vi "模字量AD输入统计结果.vi"   [LabVIEW 2010]
uses:
  全局量/自动测试结果.vi
  全局量/全局_配置.vi
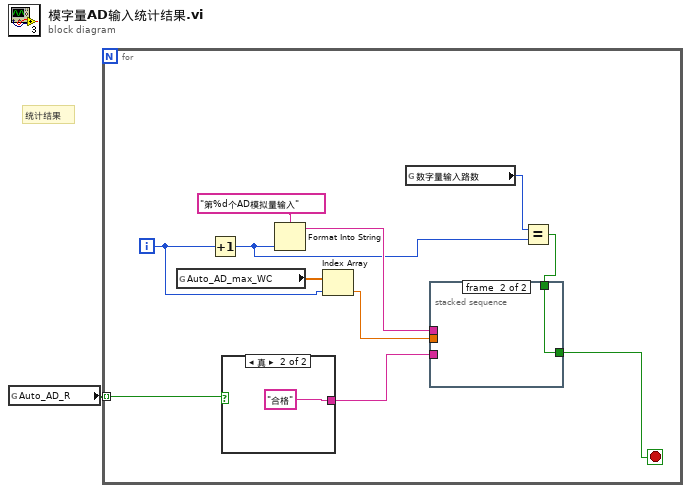
[diagram p0: block diagram]
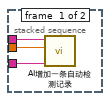
[diagram p2: hidden frame]
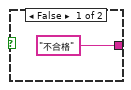
[diagram p3: hidden frame]
diagram:
  # "统计结果"
  n1 = global read "自动测试结果.vi" "Auto_AD_R"() -> (w1:bool[])
  n2 = for {
    tunnel: w1 -> [w12] mode=indexing
    i -> [w7]
    stop <- w3 stop-if-true
    n3 = global read "自动测试结果.vi" "Auto_AD_max_WC"() -> (w8:dbl[])
    n4 = Increment(x=w7) -> (x+1=w4:i32)
    n5 = case shown="真" w12 {
      tunnel: ["不合格" "合格"] -> w9
      frame False {
      }
      frame True {
      }
    }
    n6 = Format Into String(format string="第%d个AD模拟量输入", w4) -> (resulting string=w10:string)  [unwired: 2 in, 1 out]
    n7 = Index Array(array=w8, index=w7) -> (element=w6:dbl)
    n8 = global read "全局_配置.vi" "数字量输入路数"() -> (w5:i32)
    n9 = Equal?(x=w5, y=w4) -> (x = y?=w2:bool)
    n10 = stacked-sequence {
      tunnel: w10 -> [w15 _]
      tunnel: w9 -> [w14 _]
      tunnel: w6 -> [w13 _]
      tunnel: [_ w16] -> w3
      tunnel: w2 -> [_ w16]
      frame #0 {
        n11 = call "AI增加一条自动检测记录.vi"("测试结果"=w14, "最大误差"=w13, "测试内容"=w15) -> ()  [unwired: 9 in]
      }
      frame #1 {
      }
    }
  }
